vi "rad_Globals.vi"() -> ()   [LabVIEW 2016]
panel:
  in  "Global Timeout (ms)":u32=4000
  in  "RAD File Version":string="16.0.0"
  in  "Release Date":string="January 2016"
  in  "Empty List Message":string="Selected folder is empty."
  in  "RAD Wiki URL":string="http://www.ni.com/example/30986/en/"
  in  "Msg_NewerVer":string="One or more newer RAD images are present.\nPlease download the latest version of RAD from:"
  in  "Msg_OldVer":string="One or more older RAD images are present.\nPlease convert any older images by selecting \"Convert Images\" from the \"Images\" menu, then specifying either an image file or repository."
  out "ShownImageVersionDialog":bool
  out "Manager Permissions":bool=TRUE
  in  "RAD App Version":string="16.1"
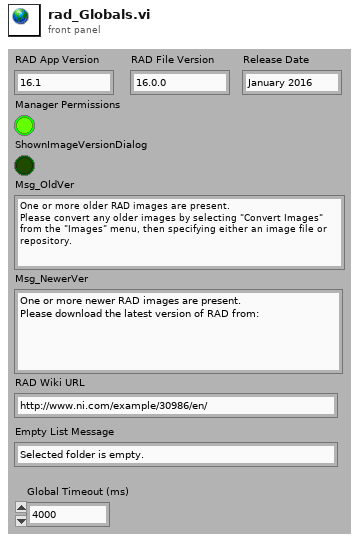
[diagram p1: front panel]
diagram:
